vi "LabVIEW datatype to Measurement datatype.vi"(8 "error in":errorcluster, 11 "type":T2) -> (0 "error out":errorcluster, 1 "Supported?":bool, 2 "Array?":bool, 3 "MessageElementType":T1)   [LabVIEW 2020, in "MeasurementTemplate_server.lvlib"]
uses:
  <vilib>/Utility/Data Type/Type Definitions/Data Type.ctl
  RPC Messages/google_protobuf_Field_Kind.ctl
  MeasurementTemplate_server.lvlib
  <vilib>/Utility/Data Type/NI_Data Type.lvlib
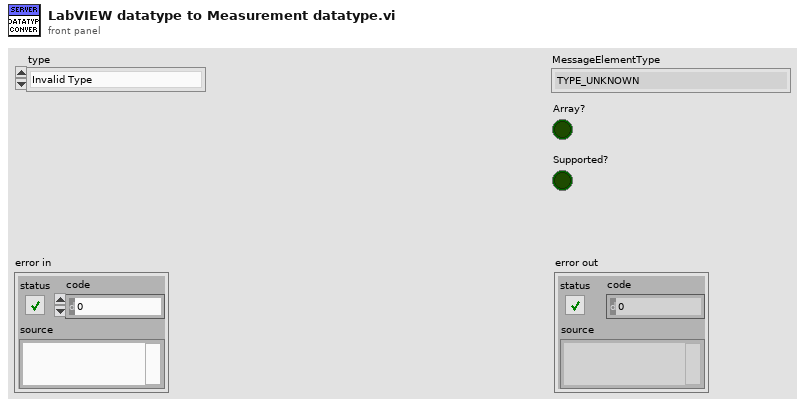
[diagram p1: front panel]
types:
  T1 = typedef "MeasurementTemplate_server.lvlib/google_protobuf_Field_Kind.ctl" = enum32{"TYPE_UNKNOWN", "TYPE_DOUBLE", "TYPE_FLOAT", "TYPE_INT64", "TYPE_UINT64", "TYPE_INT32", "TYPE_FIXED64", "TYPE_FIXED32", "TYPE_BOOL", "TYPE_STRING", "TYPE_GROUP", "TYPE_MESSAGE", "TYPE_BYTES", "TYPE_UINT32", "TYPE_ENUM", "TYPE_SFIXED32", "TYPE_SFIXED64", "TYPE_SINT32", "TYPE_SINT64"}
  T2 = typedef "NI_Data Type.lvlib/Data Type.ctl" = enum8{"Invalid Type", "Void", "I8", "I16", "I32", "I64", "U8", "U16", "U32", "U64", "Single Float", "Double Float", "Extended Float", "Single Complex", "Double Complex", "Extended Complex", "Enum U8", "Enum U16", "Enum U32", "Enum U64", "Single Float With Unit", "Double Float With Unit", "Extended Float With Unit", "Single Complex with Unit", "Double Complex with Unit", "Extended Complex with Unit", "Boolean", "String", "Path", "Picture", "Tag", "Array", "Cluster", "Variant", "LV Variant", "Waveform", "Timestamp", "Digital Waveform", "Digital Data", "ExpressData", "Refnum", "External Data", "VI", "Poly VI", "LabVIEW Class Instance", "Fixed Point", "Set Collection", "Map Collection"}
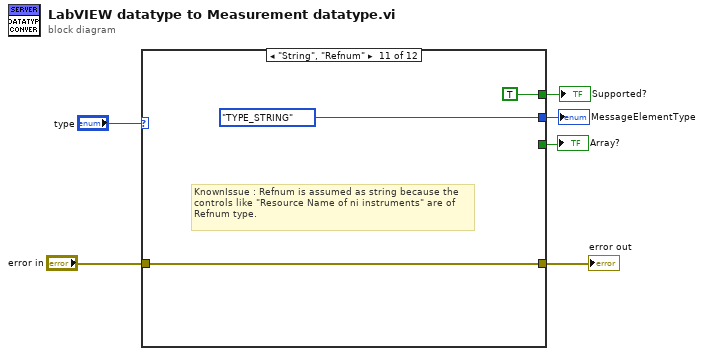
[diagram p0: block diagram]
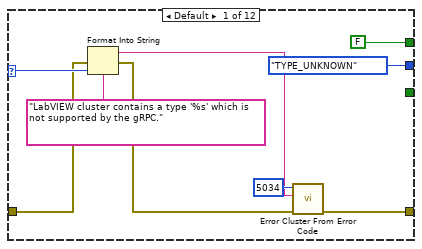
[diagram p2: hidden frame]
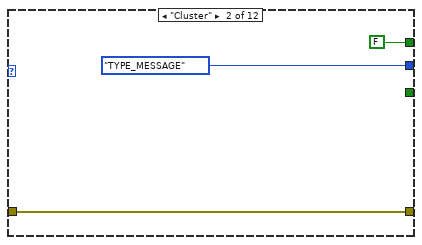
[diagram p3: hidden frame]
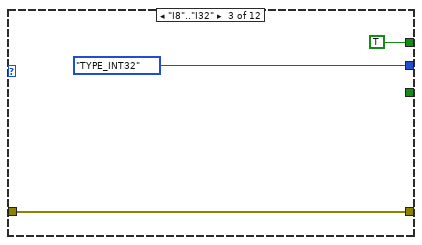
[diagram p4: hidden frame]
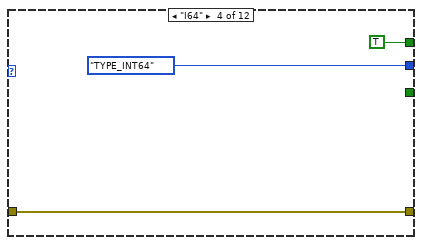
[diagram p5: hidden frame]
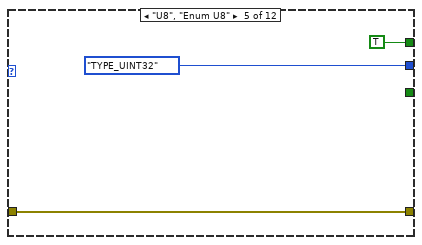
[diagram p6: hidden frame]
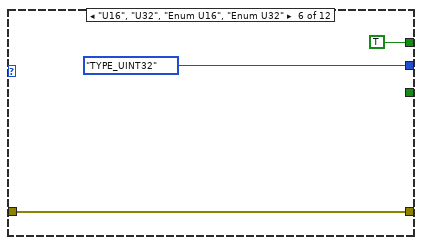
[diagram p7: hidden frame]
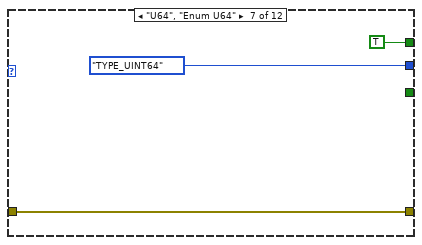
[diagram p8: hidden frame]
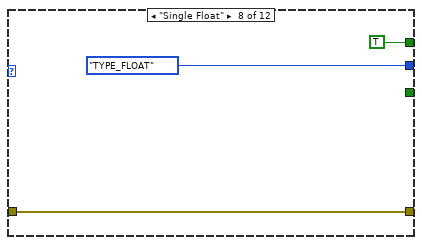
[diagram p9: hidden frame]
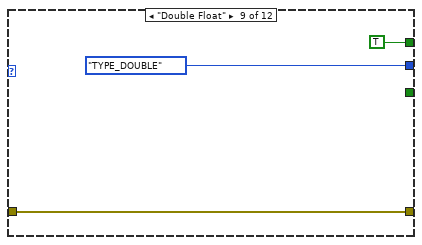
[diagram p10: hidden frame]
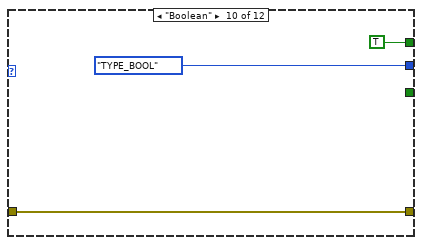
[diagram p11: hidden frame]
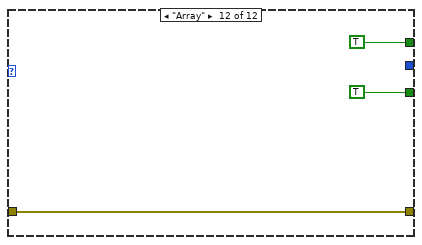
[diagram p12: hidden frame]
diagram:
  n1 = case shown="\"String\", \"Refnum\"" "type" {
    selector: "type" -> [w11 _ _ _ _ _ _ _ _ _ _ _]
    tunnel: [google_protobuf_Field_Kind."TYPE_UNKNOWN" ("MessageElementType") google_protobuf_Field_Kind."TYPE_MESSAGE" ("MessageElementType") google_protobuf_Field_Kind."TYPE_INT32" ("MessageElementType") google_protobuf_Field_Kind."TYPE_INT64" ("MessageElementType") google_protobuf_Field_Kind."TYPE_UINT32" ("MessageElementType") google_protobuf_Field_Kind."TYPE_UINT32" ("MessageElementType") google_protobuf_Field_Kind."TYPE_UINT64" ("MessageElementType") google_protobuf_Field_Kind."TYPE_FLOAT" ("MessageElementType") google_protobuf_Field_Kind."TYPE_DOUBLE" ("MessageElementType") google_protobuf_Field_Kind."TYPE_BOOL" ("MessageElementType") google_protobuf_Field_Kind."TYPE_STRING" ("MessageElementType") _] -> w5
    tunnel: [FALSE FALSE TRUE TRUE TRUE TRUE TRUE TRUE TRUE TRUE TRUE TRUE] -> w4
    tunnel: [_ _ _ _ _ _ _ _ _ _ _ TRUE] -> w3
    tunnel: "error in" -> [w7 w16 w19 w22 w25 w28 w31 w34 w37 w40 w43 w46]
    tunnel: [w13 w16 w19 w22 w25 w28 w31 w34 w37 w40 w43 w46] -> w1
    frame Default {
      n2 = Format Into String(format string="LabVIEW cluster contains a type '%s' which is not supported by the gRPC.", error in=w7, w11) -> (resulting string=w9:string, error out=w8:errorcluster)  [unwired: 1 in]
      n3 = call <vilib>:"Error Cluster From Error Code.vi"("error in (no error)"=w8, "error message (\"\")"=w9, "error code (0)"=5034) -> ("error out"=w13:errorcluster)  [unwired: 6 in]
    }
    frame "Cluster" {
    }
    frame "I8".."I32" {
    }
    frame "I64" {
    }
    frame "U8", "Enum U8" {
    }
    frame "U16", "U32", "Enum U16", "Enum U32" {
    }
    frame "U64", "Enum U64" {
    }
    frame "Single Float" {
    }
    frame "Double Float" {
    }
    frame "Boolean" {
    }
    frame "String", "Refnum" {
      # "KnownIssue : Refnum is assumed as string because the controls like \"Resource Name of ni instruments\" are of Refnum type."
    }
    frame "Array" {
    }
  }
  "MessageElementType" <- w5
  "Supported?" <- w4
  "Array?" <- w3
  "error out" <- w1
